vi "Read VI Path.vi"(9 "RasPi Compiler in":refnum<class "RasPi Compiler.lvclass">) -> (3 "RasPi Compiler out":refnum<class "RasPi Compiler.lvclass">, 4 "VI Path":path)   [LabVIEW 2014, in "Raspberry Pi Compatible Compiler for LabVIEW.lvlib" / "RasPi Compiler.lvclass"]
uses:
  RasPi Compiler.lvclass
  RasPi Compiler.lvclass/RasPi Compiler.ctl
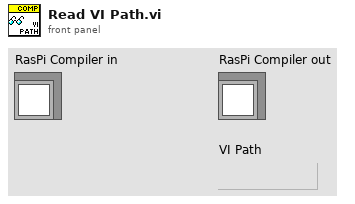
[diagram p1: front panel]
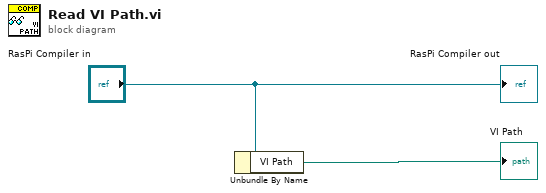
[diagram p0: block diagram]
diagram:
  n1 = Unbundle By Name("RasPi Compiler in") -> ("VI Path"=→"VI Path":path)
  "RasPi Compiler out" <- "RasPi Compiler in"
